vi "c_Msg_ToClient_2.vi"() -> (1 "Case Label":T1)   [LabVIEW 2019, in "gRPC Client Tester.lvclass"]
doc: "This VI contains a string constant containing the name of a MHL case of the Worker that owns this VI."
uses:
  gRPC Client Tester.lvclass
  <vilib>/addons/_Workers/Library/Case Label.ctl
  <vilib>/addons/_Workers/Library/Workers.lvlib
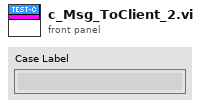
[diagram p1: front panel]
types:
  T1 = typedef "Workers.lvlib/Case Label.ctl" = string
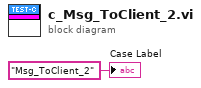
[diagram p0: block diagram]
diagram:
  "Case Label" <- T1 "Msg_ToClient_2" ("Case Label")
